vi "Error 5005 - ProtoBuf Message Was Empty.vi"() -> (0 "error out":errorcluster)   [LabVIEW 2020]
doc: "Error 5005 - ProtoBuf Message Was Empty. An attempt was made to decode a ProtoBuf message, but the ProtoBuf message was an empty string."
uses:
  <vilib>/Utility/error.llb/Error Cluster From Error Code.vi
  <vilib>/ErrorRing/Error Ring.xnode
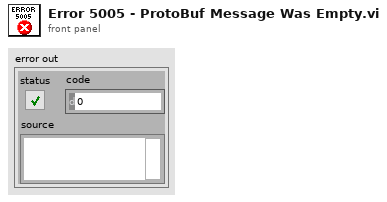
[diagram p1: front panel]
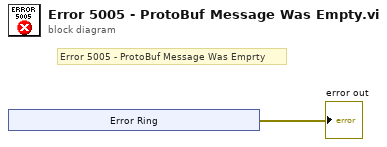
[diagram p0: block diagram]
diagram:
  # "Error 5005 - ProtoBuf Message Was Emprty"
  n1 = xnode "Error Ring"() -> ("error out"=→"error out":errorcluster)
